vi "Failing Test Cases.vi"() -> ()   [LabVIEW 2011]
uses:
  JSON Value/Set from JSON string.vi
  JSON Value/Get as JSON string.vi
  JSON Value/Get as JSON string (pretty).vi
  JSON Value/Get Item by name array.vi
  JSON Value/JSON Value.lvclass
  Get Polymorphic/JSON GetSet.lvlib
panel:
  in  "Pretty Print?":bool=TRUE
  out "Lossless":bool
  in  "JSON text that package fails on (bugs to be fixed):":string(combo)="{\"before\":1,\"Fails\":{},\"after\":1}"
  out "Unflattened and then reflattened JSON Value":string
  out "error out":errorcluster
  out "rest of JSON stream":string
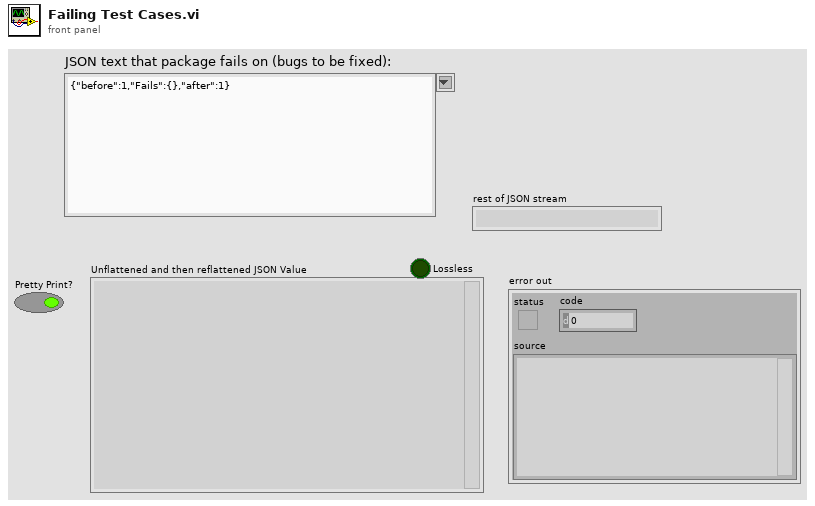
[diagram p1: front panel]
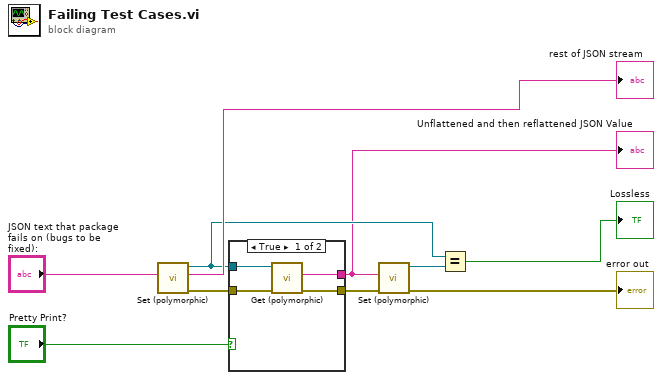
[diagram p0: block diagram]
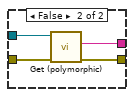
[diagram p2: hidden frame]
diagram:
  n1 = call-poly "Set (polymorphic).vi"("JSON stream"="JSON text that package fails on (bugs to be fixed):") -> ("error out"=w3:errorcluster, "rest of JSON stream"=→"rest of JSON stream":string, "JSON Value out"=w8:refnum<class "JSON Value.lvclass">)  [unwired: 8 in]
  n2 = case shown="True" "Pretty Print?" {
    tunnel: w8 -> [w14 w18]
    tunnel: [w13 w17] -> w6
    tunnel: [w12 w16] -> w4
    tunnel: w3 -> [w11 w15]
    frame True {
      n3 = call-poly "Get (polymorphic).vi"("error in (no error)"=w11, "JSON Value in"=w14) -> ("error out"=w12:errorcluster, "String"=w13:string)  [unwired: 8 in]
    }
    frame False {
      n4 = call-poly "Get (polymorphic).vi"("error in (no error)"=w15, "JSON Value in"=w18) -> ("error out"=w16:errorcluster, "String"=w17:string)  [unwired: 8 in]
    }
  }
  "Unflattened and then reflattened JSON Value" <- w6
  n5 = call-poly "Set (polymorphic).vi"("error in (no error)"=w4, "JSON stream"=w6) -> ("error out"=→"error out":errorcluster, "JSON Value out"=w7:refnum<class "JSON Value.lvclass">)  [unwired: 7 in, 1 out]
  n6 = Equal?(x=w8, y=w7) -> (x = y?=→"Lossless":bool)
